vi "Stop Watch.vi"(7 "TimerAction(Read)":T1(ring)=enum."ReadTimer", 8 "error in (no error)":errorcluster) -> (0 "error out":errorcluster, 2 "TimeLapsed(mS)":dbl)   [LabVIEW 2023, in "GUI.lvlib" / "Diagnostic.lvlib" / "VAL_SW_Testing.lvlib"]
uses:
  VAL_SW_Testing.lvlib
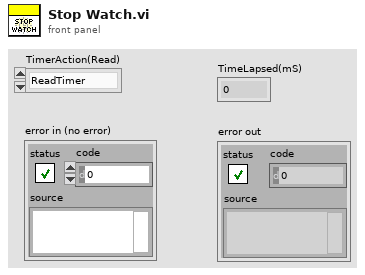
[diagram p1: front panel]
types:
  T1 = enum16{"StartTimer", "ReadTimer", "StopTimer", "Init"}
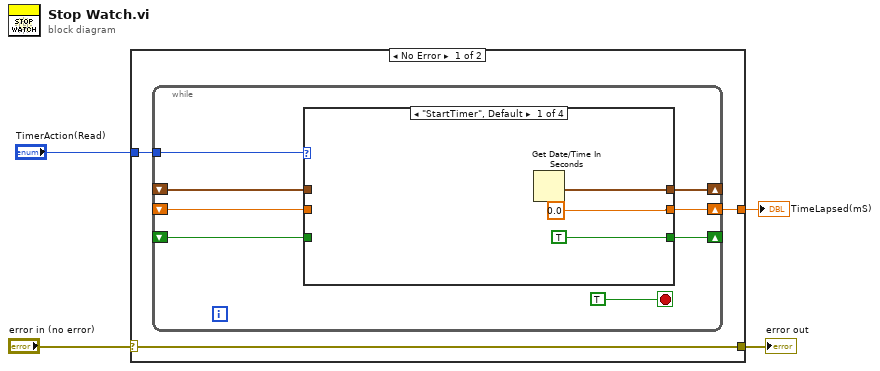
[diagram p0: block diagram]
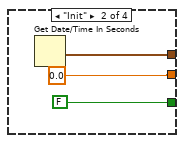
[diagram p2: hidden frame]
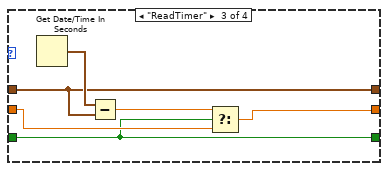
[diagram p3: hidden frame]
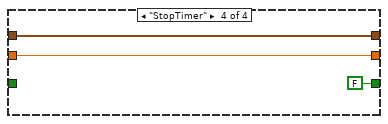
[diagram p4: hidden frame]
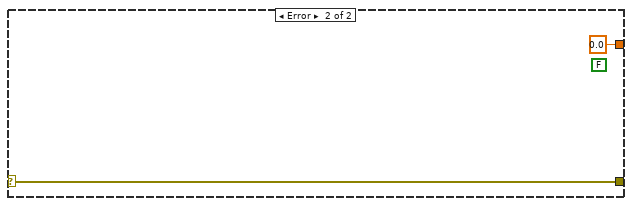
[diagram p5: hidden frame]
diagram:
  n1 = case shown="No Error" "error in (no error)" {
    selector: "error in (no error)" -> [w7 w32]
    tunnel: [w7 w32] -> w3
    tunnel: "TimerAction(Read)" -> [w6 _]
    tunnel: [w5 0.0] -> w1
    frame No Error {
      n2 = while {
        tunnel: w6 -> [w14]
        shift-right: [w13] -> _
        shift-left: _ -> [w12]
        shift-right: [w11] -> w5
        shift-left: _ -> [w10]
        shift-right: [w9] -> _
        shift-left: _ -> [w8]
        stop <- TRUE stop-if-true
        n3 = case shown="\"StartTimer\", Default" w14 {
          tunnel: [w18 w21 w26 w29] -> w13
          tunnel: w12 -> [_ _ w26 w29]
          tunnel: [0.0 0.0 w23 w30] -> w11
          tunnel: w10 -> [_ _ w24 w30]
          tunnel: [TRUE FALSE w22 FALSE] -> w9
          tunnel: w8 -> [_ _ w22 _]
          frame "StartTimer", Default {
            n4 = Get Date/Time In Seconds() -> (seconds since 1Jan1904=w18:timestamp)
          }
          frame "Init" {
            n5 = Get Date/Time In Seconds() -> (seconds since 1Jan1904=w21:timestamp)
          }
          frame "ReadTimer" {
            n6 = Get Date/Time In Seconds() -> (seconds since 1Jan1904=w27:timestamp)
            n7 = Subtract(x=w27, y=w26) -> (x-y=w25:dbl)
            n8 = Select(t=w25, s=w22, f=w24) -> (s? t:f=w23:dbl)
          }
          frame "StopTimer" {
          }
        }
      }
    }
    frame Error {
      (unwired) FALSE
    }
  }
  "error out" <- w3
  "TimeLapsed(mS)" <- w1
